vi "convert lines.vi"(10 "lines[]":cluster{"y":i32, "x start":i32, "x end":i32}[](array[cluster])) -> (1 "rect":T1, 3 "array (x start, x length)":cluster{i32, i32}[](array[cluster]))   [LabVIEW 2009]
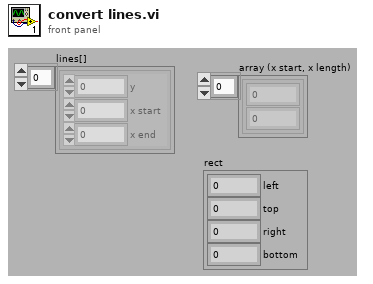
[diagram p1: front panel]
types:
  T1 = cluster{"left":i16, "top":i16, "right":i16, "bottom":i16}
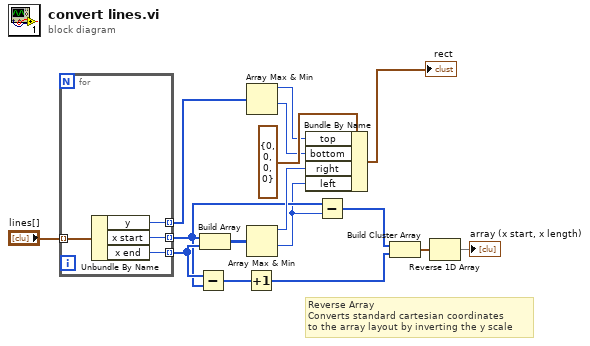
[diagram p0: block diagram]
diagram:
  # "Reverse Array\nConverts standard cartesian coordinates\nto the array layout by inverting the y scale"
  n1 = for {
    tunnel: "lines[]" -> [w20] mode=indexing
    tunnel: [w19] -> w6 mode=indexing
    tunnel: [w18] -> w8 mode=indexing
    tunnel: [w17] -> w15 mode=indexing
    n2 = Unbundle By Name(w20) -> ("y"=w17:i32, "x start"=w19:i32, "x end"=w18:i32)
  }
  n3 = Subtract(x=w8, y=w6) -> (x-y=w7:i32[])
  n4 = Build Array(w6, w8) -> (w16:i32[][])
  n5 = Increment(x=w7) -> (x+1=w3:i32[])
  n6 = Array Max & Min(array=w15) -> (max value=w13:i32, min value=w12:i32)  [unwired: 2 out]
  n7 = Array Max & Min(array=w16) -> (max value=w11:i32, min value=w5:i32)  [unwired: 2 out]
  n8 = Bundle By Name(cluster=T1 {"left"=0, "top"=0, "right"=0, "bottom"=0} ("rect"), "top"=w13, "bottom"=w12, "right"=w11, "left"=w5) -> (→"rect":T1)
  n9 = Subtract(x=w6, y=w5) -> (x-y=w4:i32[])
  n10 = Build Cluster Array(w4, w3) -> (w2:cluster{i32, i32}[])
  n11 = Reverse 1D Array(array=w2) -> (reversed array=→"array (x start, x length)":cluster{i32, i32}[])
